vi "Goal Pose.vi"() -> ()   [LabVIEW 2016]
panel:
  in  "Pose":dbl[](array[numeric])
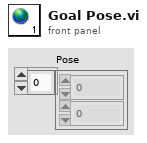
[diagram p1: front panel]
diagram:
